vi "LED - Pin Cycle through all Pixels.vi"   [LabVIEW 2015]
doc: "This example demonstrates a rainbow effect on a 1-wire RGB LED strip using a WS2811 or WS2812 controller. Each LED in the strip is gradually changed from red to green, then to blue with a blend of colors in between. The LED color changing effect is staggered down the strip so not all LEDs are changed at the same time. The time delay can also be adjusted to change how fast the color is changed."
uses:
  <vilib>/Aledyne-TSXperts/Arduino Compatible Compiler for LabVIEW/Code Generator/Arduino APIs/RGB LED Strip/RGB Strip Mode.ctl
  <vilib>/Aledyne-TSXperts/Arduino Compatible Compiler for LabVIEW/Arduino Compatible Compiler for LabVIEW.lvlib
panel:
  # "Overview: Demonstrates a rainbow effect on a 1-wire RGB LED strip using a WS2811 or WS2812 controller.  Each LED in the strip is gradually changed from red to green, then to blue with a blend of colors in between.  The LED color changing effect is staggered down the strip so not all LEDs are changed at the same time.  The time delay can also be adjusted to change how fast the color is changed.\n\nInstructions:\n1. Wire a 1-wire LED strip to a digital pin on the Arduino board.  Follow wiring instructions from the manufacturer.  A 100-500 ohm resistor is usually recommended between the Arduino digital output and the LED strip's data in pin.  Also, a 100 uF capacitor between the ground and power input may reduce noise on from the power supply.  It is also recommended to power the LED strip from a separate power input if available on the strip.  When daisy chaining LED strips, it is recommended to only daisy chain the Data line and to power each strip from a separate power input.\n2. Set the Digital Pin wired below.\n3. Set the Mode to the correct setting for your LED strip (the WS2812 uses 800kHz GRB).\n4. Set the Number of LEDs on your strip.  This can be set to any number equal to or smaller than the number of physical LEDs on the strip of you do not wish to power up all of them.\n5. Set the delay (ms) between changes to the LED color.\n6.  If this example has been loaded from the Arduino Compatible Compiler for LabVIEW, simply select Compile and Download.  Otherwise, open Tools>Arduino Compatible Compiler for LabVIEW in LabVIEW, then select File>Load VI, and select this VI and then Compile and Download.\n7. Observe the LEDs on the strip changing color with a seamless rainbow transition."
types:
  T1 = typedef "Arduino Compatible Compiler for LabVIEW.lvlib/RGB Strip Mode.ctl" = u16
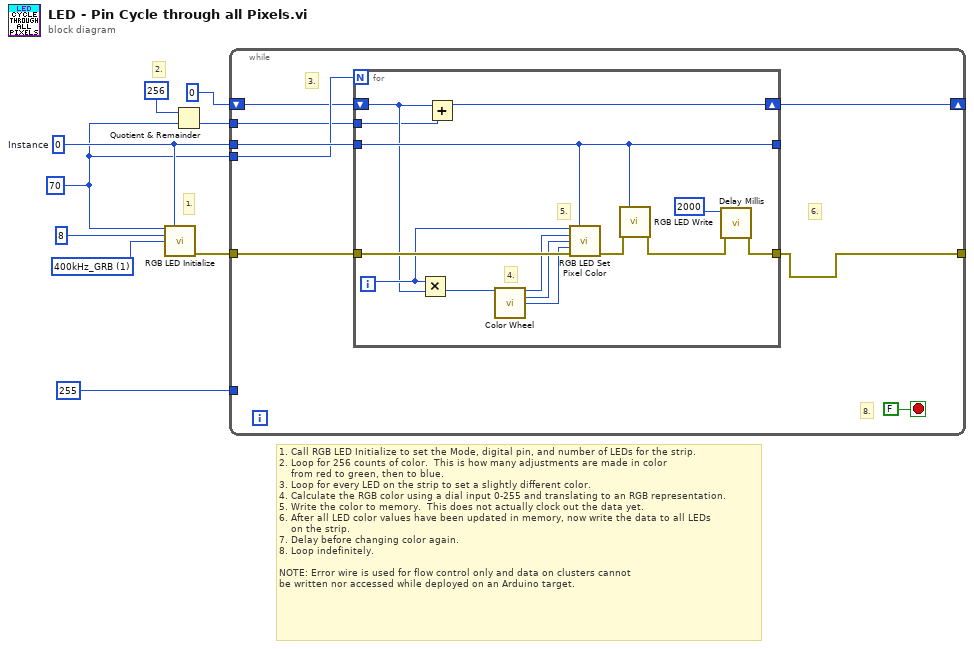
[diagram p0: block diagram]
diagram:
  w3 = u16 70 ("Number of LEDs")
  w9 = T1 1 items=["400kHz_RGB"=0, "400kHz_GRB"=1, "400kHz_BRG"=4, "800kHz_RGB"=2, "800kHz_GRB"=3, "400kHz_BRG"=6] ("Mode")
  w6 = u8 0  # Instance
  # "2."
  # "1."
  # "1. Call RGB LED Initialize to set the Mode, digital pin, and number of LEDs for the strip.\n2. Loop for 256 counts of color.  This is how many adjustments are made in color\n    from red to green, then to blue.\n3. Loop for every LED on the strip to set a slightly different color.\n4. Calculate the RGB color using a dial input 0-255 and translating to an RGB representation.\n5. Write the color to memory.  This does not actually clock out the data yet.\n6. After all LED color values have been updated in memory, now write the data to all LEDs\n    on the strip.\n7. Delay before changing color again.\n8. Loop indefinitely.\n\nNOTE: Error wire is used for flow control only and data on clusters cannot\nbe written nor accessed while deployed on an Arduino target."
  n1 = call <vilib>:"RGB LED Initialize.vi"("Number of Pixels"=w3, "Instance"=w6, "Pin"=u8 8 ("Digital Pin"), "Mode"=w9) -> ("error out"=w7:errorcluster)  [unwired: 11 in]
  n2 = Quotient & Remainder(x=u16 256 ("Number of Pixels"), y=w3) -> (floor(x/y)=w1:u16)  [unwired: 1 out]
  n3 = while {
    tunnel: w7 -> [w16]
    tunnel: w6 -> [w15]
    tunnel: w3 -> [w14]
    tunnel: u8 255 ("delay (ms)") -> [_]
    tunnel: [w13] -> _
    shift-right: [w10] -> _
    shift-left: u16 0 ("floor(x/y)") -> [w12]
    tunnel: w1 -> [w11]
    stop <- FALSE stop-if-true
    # "6."
    # "3."
    # "8."
    n4 = for {
      N: w14 -> [_]
      tunnel: w15 -> [w21]
      tunnel: w16 -> [w31]
      tunnel: [w25] -> w13
      tunnel: [w21] -> _
      shift-right: [w18] -> w10
      shift-left: w12 -> [w20]
      tunnel: w11 -> [w19]
      i -> [w27]
      # "5."
      # "4."
      n5 = Multiply(x=w27, y=w20) -> (x*y=w26:i32)
      n6 = Add(x=w20, y=w19) -> (x+y=w18:u16)
      n7 = call "Color Wheel.vi"("Dial Position"=w26) -> ("Red"=w30:u8, "Green"=w29:u8, "Blue"=w28:u8)  [unwired: 12 in]
      n8 = call <vilib>:"RGB LED Set Pixel Color.vi"("Pixel"=w27, "Instance"=w21, "Red"=w30, "Green"=w29, "Blue"=w28, "error in (no error)"=w31) -> ("error out"=w23:errorcluster)  [unwired: 9 in]
      n9 = call <vilib>:"RGB LED Write.vi"("Instance"=w21, "error in (no error)"=w23) -> ("error out"=w22:errorcluster)  [unwired: 13 in]
      n10 = call <vilib>:"Delay Millis.vi"("error in (no error)"=w22, "delay"=u32 2000) -> ("error out"=w25:errorcluster)  [unwired: 9 in]
    }
  }
